vi "Get Configuration File Target Path.vi"(8 "error in (no error)":errorcluster, 11 "Item Ref in":T1 format="%.0x") -> (0 "error out":errorcluster, 2 "configuration target path":path, 3 "Item Ref out":T1 format="%.0x")   [LabVIEW 2020, in "DSF Shared.lvlib"]
uses:
  DSF Shared.lvlib
  <vilib>/NI VeriStand/Custom Device API/Custom Device Item Ref.ctl
  <vilib>/NI VeriStand/Custom Device API/Get Item Property (Path).vi
  <vilib>/NI VeriStand/Custom Device API/Custom Device API.lvlib
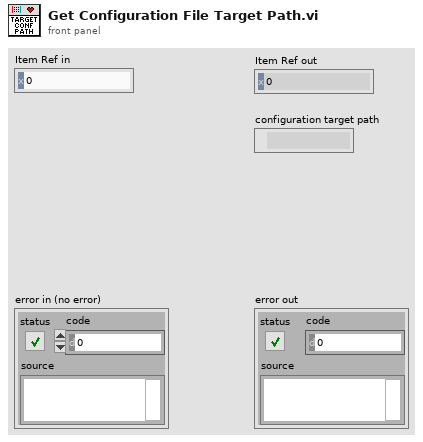
[diagram p1: front panel]
types:
  T1 = typedef "Custom Device API.lvlib/Custom Device Item Ref.ctl" = u64
  T2 = typedef "Custom Device API.lvlib/Custom Device Target Type.ctl" = enum16{"PharLap", "VxWorks", "Windows", "Linux_32_ARM", "Linux_x64"}
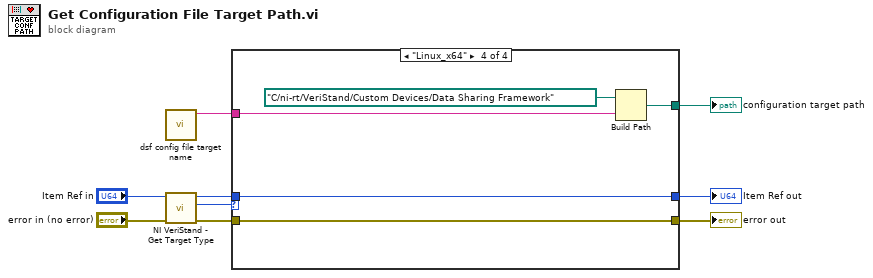
[diagram p0: block diagram]
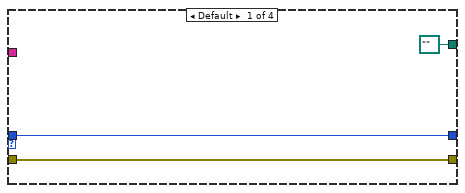
[diagram p2: hidden frame]
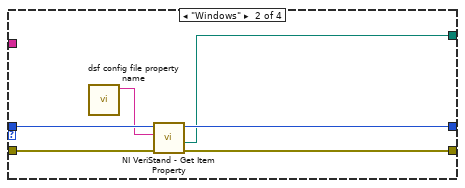
[diagram p3: hidden frame]
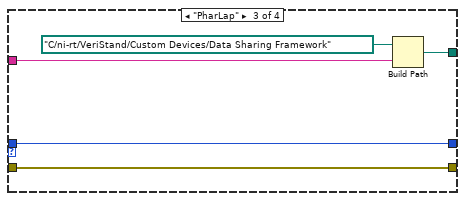
[diagram p4: hidden frame]
diagram:
  n1 = call "dsf config file target name.vi"() -> ("config file target name"=w1:string)  [unwired: 11 in]
  n2 = call <vilib>:"NI VeriStand - Get Target Type.vi"("error in (no error)"="error in (no error)", "Item Ref in"="Item Ref in") -> ("error out"=w5:errorcluster, "Target Type"=w7:T2, "Item Ref out"=w6:T1)  [unwired: 7 in]
  n3 = case shown="\"Linux_x64\"" w7 {
    tunnel: w6 -> [w12 w18 w19 w24]
    tunnel: w5 -> [w11 w17 w20 w25]
    tunnel: w1 -> [_ _ w22 w27]
    tunnel: [path "" ("appended path") w14 w21 w26] -> w4
    tunnel: [w11 w15 w20 w25] -> w3
    tunnel: [w12 w16 w19 w24] -> w2
    frame Default {
    }
    frame "Windows" {
      n4 = call "dsf config file property name.vi"() -> ("file path property name"=w13:string)  [unwired: 11 in]
      n5 = call-poly <vilib>:"NI VeriStand - Get Item Property.vi"("error in (no error)"=w17, "Property Name"=w13, "Item Ref in"=w18) -> ("error out"=w15:errorcluster, "Value"=w14:path, "Item Ref out"=w16:T1)  [unwired: 5 in, 1 out]
    }
    frame "PharLap" {
      n6 = Build Path(base path=path "C:/ni-rt/VeriStand/Custom Devices/Data Sharing Framework" ("RT Destination"), name or relative path=w22) -> (appended path=w21:path)
    }
    frame "Linux_x64" {
      n7 = Build Path(base path=path "C:/ni-rt/VeriStand/Custom Devices/Data Sharing Framework" ("RT Destination"), name or relative path=w27) -> (appended path=w26:path)
    }
  }
  "Item Ref out" <- w2
  "error out" <- w3
  "configuration target path" <- w4
